vi "INI read LO sources.vi"(8 "error in (no error)":T2) -> (0 "error out":T2, 3 "data":T1={"RX/LO1 src"="Internal", "TX/LO1 src"="Internal", "LO2 src"="Internal"})   [LabVIEW 2019, in "Shared.lvlib"]
doc: "Read mmWave LO sources from ini file.\nreturns sources for TX/LO1, RX/LO1 and LO2"
uses:
  Shared.lvlib
  mmWave HW Control/LO sources.ctl
  Low-level/TypeDefs/TX trigger config.ctl
  FPGA/SubVIs/Utility/FPGA driver trigger source.ctl
  FPGA/SubVIs/Utility/FPGA driver trigger destination.ctl
  System GV.vi
  <vilib>/Utility/config.llb/NI_LVConfig.lvlib
  FPGA/SubVIs/Utility/FPGA Utility.lvlib
  mmWave HW Control/mmWave HW Control.lvlib
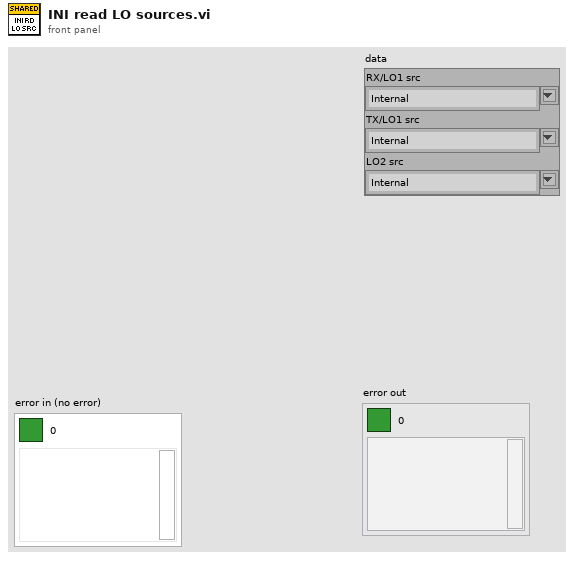
[diagram p1: front panel]
types:
  T1 = typedef "mmWave HW Control.lvlib/LO sources.ctl" = cluster{"RX/LO1 src":string, "TX/LO1 src":string, "LO2 src":string}
  T2 = cluster{"Boolean Round":bool, "code":i32, "source":string}
  T3 = typedef "TX trigger config.ctl" = cluster{"delay":dbl, "trig source":T4, "PXI src":i32, "export":T5, "PXI dest":i32}
  T4 = typedef "FPGA Utility.lvlib/FPGA driver trigger source.ctl" = enum16{"Use Tclk", "PXI_Trig", "Aurora RX trig"}
  T5 = typedef "FPGA Utility.lvlib/FPGA driver trigger destination.ctl" = enum16{"None", "Source trig", "Synced trig", "Delayed sync"}
  T6 = typedef "NI_LVConfig.lvlib/Config Data RefNum.ctl" = refnum<k1>
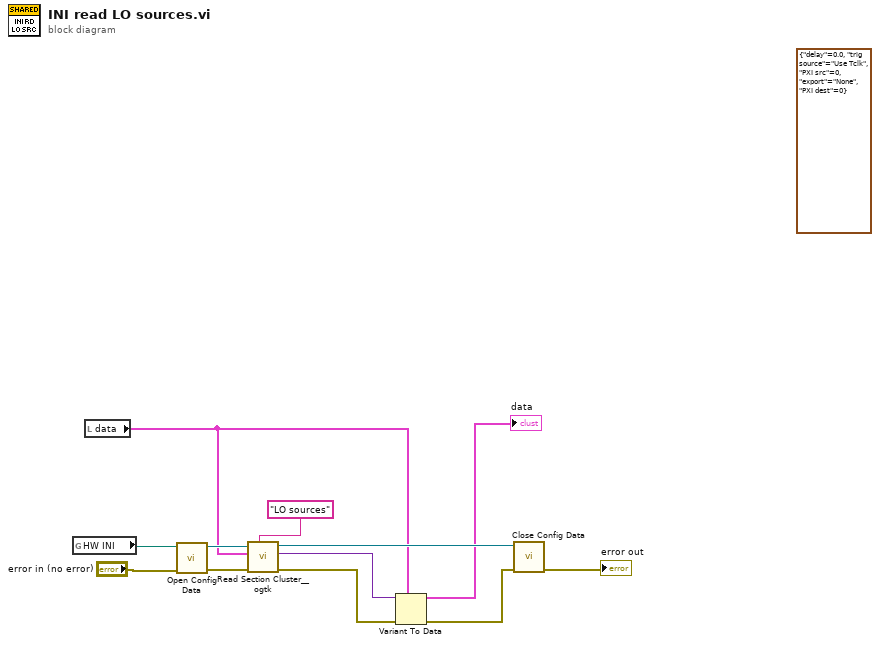
[diagram p0: block diagram]
diagram:
  (unwired) T3 {"delay"=0.0, "trig source"=enum."Use Tclk", "PXI src"=0, "export"=enum."None", "PXI dest"=0} ("TX trigger options")
  n1 = global read "System GV.vi" "HW INI"() -> (w9:path)
  n2 = local read "data"() -> (w1:T1)
  n3 = call <vilib>:"Open Config Data.vi"("error in (no error)"="error in (no error)", "configuration file path"=w9) -> ("error out"=w10:errorcluster, "refnum"=w12:T6)  [unwired: 7 in, 1 out]
  n4 = call <userlib>:"Read Section Cluster__ogtk.vi"("section (optional)"="LO sources", "error in (no error)"=w10, "Section Formatted Cluster Type"=w1, "refnum"=w12) -> ("error out"=w6:errorcluster, "Section Formatted Cluster"=w7:variant, "dup refnum"=w11:T6)  [unwired: 3 in, 2 out]
  n5 = Variant To Data(error in=w6, type=w1, Variant=w7) -> (data=→"data":T1, error out=w5:errorcluster)
  n6 = call <vilib>:"Close Config Data.vi"("error in (no error)"=w5, "refnum"=w11) -> ("error out"=→"error out":errorcluster)  [unwired: 8 in, 1 out]
